vi "Synth Init DAQ Port.vi"(4 "Use hardware clock for DO":bool=TRUE, 6 "DO Samples per Channel":i32=10000, 7 "DO Clock Rate (Hz)":dbl=500000.0, 8 "error in (no error)":errorcluster, 9 "Clock source":tag, 10 "DAQmx Device Name":tag="6251") -> (0 "error out":errorcluster, 3 "task out":refnum<k21>)   [LabVIEW 2021]
uses:
  <vilib>/DAQmx/create/channels.llb/DAQmx Create Channel (DO-Digital Output).vi
  <vilib>/DAQmx/configure/timing.llb/DAQmx Timing (Sample Clock).vi
  <resource>/objmgr/daqmx.rc
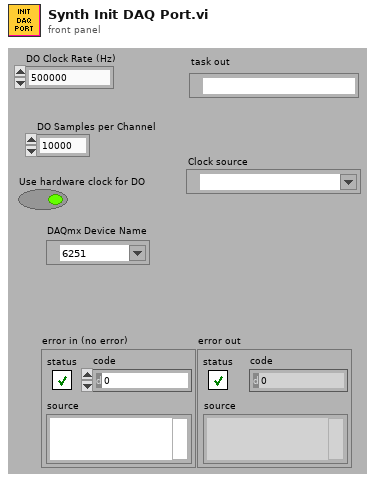
[diagram p1: front panel]
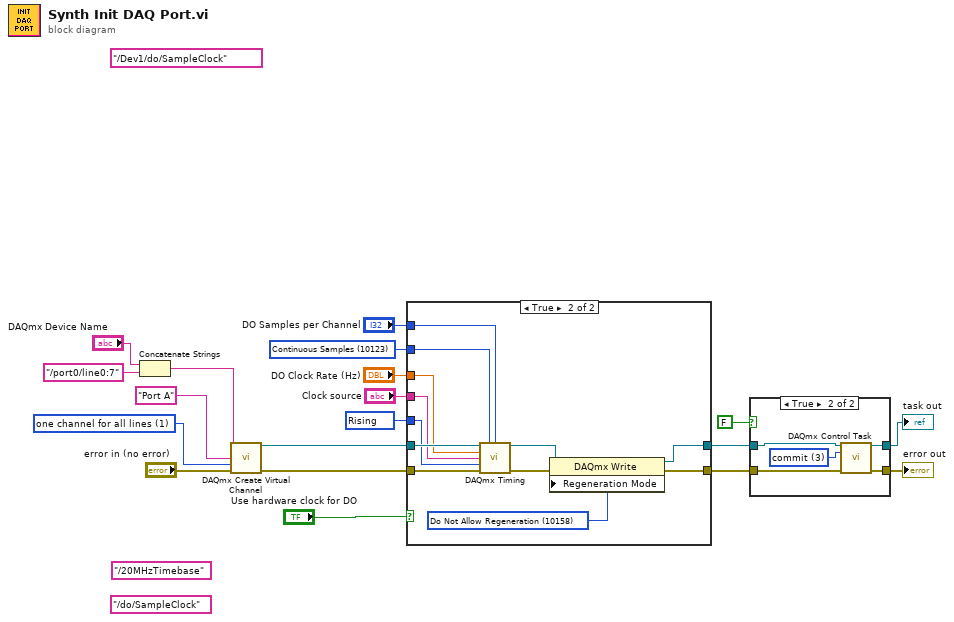
[diagram p0: block diagram]
diagram:
  (unwired) "/do/SampleClock"
  (unwired) "/20MHzTimebase"
  w12 = 10280 items=["Rising"=10280, "Falling"=10171] ("active edge")
  (unwired) tag "/Dev1/do/SampleClock" ("source")
  w13 = 1 items=["one channel for each line", "one channel for all lines"] ("line grouping")
  w17 = 10123 items=["Finite Samples"=10178, "Continuous Samples"=10123] ("sample mode")
  n1 = Concatenate Strings("DAQmx Device Name", "/port0/line0:7") -> (w7:string)
  n2 = call-poly <vilib>:"DAQmx Create Virtual Channel.vi"("lines"=w7, "name to assign"="Port A", "line grouping"=w13, "error in"="error in (no error)") -> ("task out"=w14:refnum<k21>, "error out"=w15:errorcluster)  [unwired: 1 in, 9 out]
  n3 = case shown="True" "Use hardware clock for DO" {
    tunnel: "DO Samples per Channel" -> [_ w33]
    tunnel: [w20 w25] -> w18
    tunnel: w17 -> [_ w32]
    tunnel: w15 -> [w21 w31]
    tunnel: w14 -> [w20 w30]
    tunnel: w12 -> [_ w29]
    tunnel: "DO Clock Rate (Hz)" -> [_ w28]
    tunnel: [w21 w22] -> w3
    tunnel: "Clock source" -> [_ w27]
    frame False {
    }
    frame True {
      w24 = 10158 items=["Allow Regeneration"=10097, "Do Not Allow Regeneration"=10158] ("RegenMode")
      n4 = call-poly <vilib>:"DAQmx Timing.vi"("task/channels in"=w30, "sample mode"=w32, "samples per channel"=w33, "rate"=w28, "source"=w27, "active edge"=w29, "error in"=w31) -> ("task out"=w26:refnum<k21>, "error out"=w23:errorcluster)  [unwired: 7 out]
      n5 = property class="DAQmx Write"(reference=w26, error in=w23, "Regeneration Mode"=w24) -> (reference out=w25:refnum<k21>, error out=w22:errorcluster)
    }
  }
  n6 = case shown="True" FALSE {
    tunnel: w18 -> [w35 w40]
    tunnel: [w35 w39] -> w4
    tunnel: w3 -> [w34 w37]
    tunnel: [w34 w36] -> w2
    frame False {
    }
    frame True {
      w38 = 3 items=["verify"=2, "reserve"=4, "commit"=3, "unreserve"=5, "abort"=6] ("action")
      n7 = call <vilib>:"DAQmx Control Task.vi"("task/channels in"=w40, "action"=w38, "error in"=w37) -> ("task out"=w39:refnum<k21>, "error out"=w36:errorcluster)  [unwired: 11 out]
    }
  }
  "task out" <- w4
  "error out" <- w2
